vi "Digital - Continuous Input.vi"() -> ()   [LabVIEW 2014]
doc: "This example demonstrates how to acquire a continuous amount of digital data based off of a sample clock.\n\nSome hardware (e.g. M Series DAQ) must use an external sample clock for digital tasks. To view a complete list of available sample clock sources, consult the Device Routes table in Measurement and Automation Explorer.\n\nFor instructions on how to connect your signals to the DAQ device, refer to your device documentation."
uses:
  <vilib>/Utility/error.llb/DialogType.ctl
  <vilib>/DAQmx/read.llb/DAQmx Read (Digital Wfm 1Chan NSamp).vi
  <vilib>/DAQmx/create/channels.llb/DAQmx Create Channel (DI-Digital Input).vi
  <vilib>/DAQmx/configure/timing.llb/DAQmx Timing (Sample Clock).vi
  <vilib>/DAQmx/configure/trigger.llb/DAQmx Start Trigger (Digital Edge).vi
  <vilib>/DAQmx/configure/trigger.llb/DAQmx Reference Trigger (Digital Edge).vi
  <vilib>/DAQmx/miscellaneous.llb/DAQmx Fill In Error Info.vi
  <vilib>/Waveform/DWDTOps.llb/DWDT Digital to Binary U8.vi
  <resource>/objmgr/daqmx.rc
panel:
  in  "write to disk":bool
  in  "file path (use dialog)":path=path "e:/fire3.dat"
  in  "Samples per Loop":i32=100000
  in  "Stop":bool
  out "Digital Waveform Graph":digitalwaveform(graph)
  in  "Trigger Type":T1(tab)=enum."Digital Start"
  in  "Edge":i32(ring)=10280 items=["Rising"=10280, "Falling"=10171]
  in  "Digital Trigger Source":tag="/Dev1/PFI9"
  in  "Digital Trigger Source":tag="/Dev1/PFI9"
  in  "Edge":i32(ring)=10280 items=["Rising"=10280, "Falling"=10171]
  in  "pretrigger samples per channel":u32=2
  in  "Sample Rate":dbl=100000.0
  in  "Sample Clock Source":tag="OnboardClock"
  out "Actual Sample Rate":dbl=1000.0 format="%0.2f"
  in  "Line(s)":tag="Dev1/port0/line0:2"
  # "Channel Settings"
  # "Acquired Data"
  # "Timing Settings"
  # "Logging Settings"
  # "Trigger Settings"
  # "To configure and use a start trigger you must have the necessary tab selected above.  Not all hardware supports triggering--refer to your device documentation for more info."
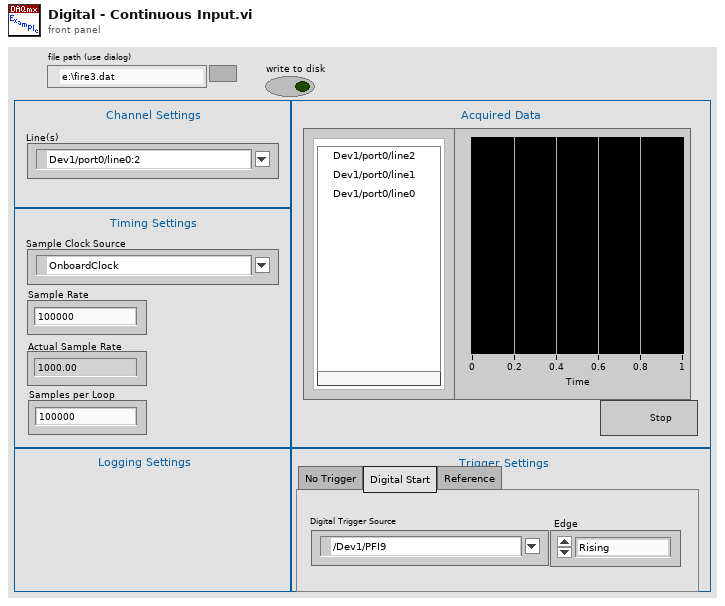
[diagram p1: front panel]
types:
  T1 = enum32{"No Trigger", "Digital Start", "Reference"}
  T2 = typedef "DialogType.ctl" = u16
  T3 = enum16{"big-endian, network order", "native, host order", "little-endian"}
  T4 = enum16{"open", "replace", "create", "open or create", "replace or create", "replace or create with confirmation"}
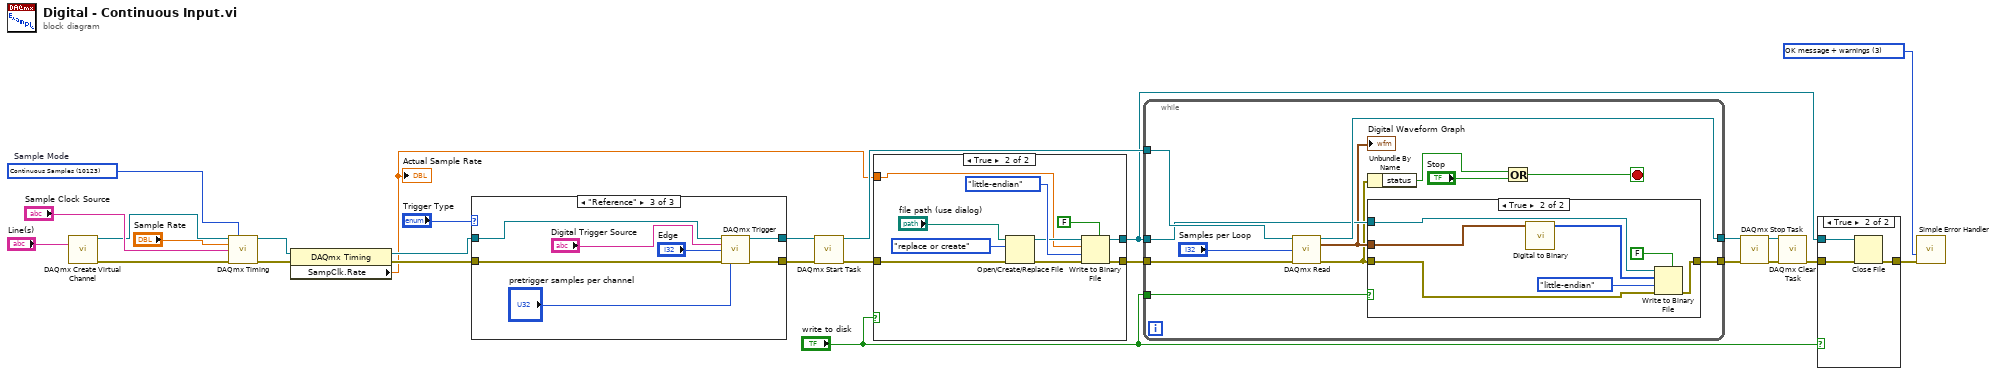
[diagram p0: block diagram]
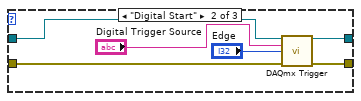
[diagram p6: hidden frame]
diagram:
  w10 = T2 3 items=["no dialog", "OK message", "continue or stop message", "OK message + warnings", "continue/stop + warnings"] ("type of dialog (OK msg:1)")
  w25 = 10123 items=["Finite Samples"=10178, "Continuous Samples"=10123, "Hardware Timed Single Point"=12522]  # Sample Mode
  n1 = call-poly <vilib>:"DAQmx Create Virtual Channel.vi"("lines"="Line(s)") -> ("task out"=w22:refnum<k21>, "error out"=w21:errorcluster)  [unwired: 13 in]
  n2 = call-poly <vilib>:"DAQmx Timing.vi"("task/channels in"=w22, "sample mode"=w25, "rate"="Sample Rate", "source"="Sample Clock Source", "error in"=w21) -> ("task out"=w20:refnum<k21>, "error out"=w19:errorcluster)  [unwired: 9 in]
  n3 = property class="DAQmx Timing"(reference=w20, error in=w19) -> (reference out=w8:refnum<k21>, error out=w9:errorcluster, "SampClk.Rate"=w1:dbl)
  "Actual Sample Rate" <- w1
  n4 = case shown="\"Reference\"" "Trigger Type" {
    tunnel: w8 -> [w28 w34 w41]
    tunnel: w9 -> [w27 w33 w40]
    tunnel: [w28 w32 w39] -> w17
    tunnel: [w27 w31 w38] -> w16
    frame "No Trigger", Default {
    }
    frame "Digital Start" {
      n5 = call-poly <vilib>:"DAQmx Trigger.vi"("task/channels in"=w34, "source"="Digital Trigger Source", "edge"="Edge", "error in"=w33) -> ("task out"=w32:refnum<k21>, "error out"=w31:errorcluster)  [unwired: 10 in]
    }
    frame "Reference" {
      n6 = call-poly <vilib>:"DAQmx Trigger.vi"("task/channels in"=w41, "source"="Digital Trigger Source", "edge"="Edge", "error in"=w40, "pretrigger samples per channel"="pretrigger samples per channel") -> ("task out"=w39:refnum<k21>, "error out"=w38:errorcluster)  [unwired: 9 in]
    }
  }
  n7 = call <vilib>:"DAQmx Start Task.vi"("task/channels in"=w17, "error in"=w16) -> ("task out"=w15:refnum<k21>, "error out"=w4:errorcluster)  [unwired: 12 in]
  n8 = case shown="True" "write to disk" {
    tunnel: [_ w46] -> w5
    tunnel: w4 -> [w42 w50]
    tunnel: [w42 w44] -> w3
    tunnel: w1 -> [_ w43]
    frame False {
    }
    frame True {
      n9 = Open/Create/Replace File(file path (use dialog)="file path (use dialog)", error in=w50, operation (0:open)=T4."replace or create") -> (refnum out=w47:refnum<file>, error out=w45:errorcluster)  [unwired: 3 in, 1 out]
      n10 = Write to Binary File(file (use dialog)=w47, data=w43, error in=w45, 5:FALSE ("prepend array or string size? (T)"), 9:T3."little-endian" ("byte order (0:big-endian, network order)")) -> (refnum out=w46:refnum<file>, error out=w44:errorcluster)  [unwired: 1 in, 1 out]
    }
  }
  n11 = while {
    tunnel: [w64] -> w12
    tunnel: [w54] -> w11
    tunnel: w3 -> [w63]
    tunnel: w15 -> [w62]
    tunnel: w5 -> [w57]
    tunnel: "write to disk" -> [w53]
    stop <- w59 stop-if-true
    n12 = call-poly <vilib>:"DAQmx Read.vi"("task/channels in"=w62, "number of samples per channel"="Samples per Loop", "error in"=w63) -> ("task out"=w64:refnum<k21>, "data"=w56:digitalwaveform, "error out"=w55:errorcluster)  [unwired: 10 in]
    "Digital Waveform Graph" <- w56
    n13 = Unbundle By Name(w55) -> ("status"=w61:bool)
    n14 = case shown="True" w53 {
      tunnel: w57 -> [_ w67]
      tunnel: w56 -> [_ w72]
      tunnel: w55 -> [w65 w66]
      tunnel: [w65 w70] -> w54
      frame False {
      }
      frame True {
        n15 = call-poly <vilib>:"Digital to Binary.vi"("digital waveform"=w72) -> ("binary array"=w71:u8[])  [unwired: 9 in, 1 out]
        n16 = Write to Binary File(file (use dialog)=w67, data=w71, error in=w66, 5:FALSE ("prepend array or string size? (T)"), 9:T3."little-endian" ("byte order (0:big-endian, network order)")) -> (error out=w70:errorcluster)  [unwired: 1 in, 2 out]
      }
    }
    n17 = Or(x=w61, y="Stop") -> (x .or. y?=w59:bool)
  }
  n18 = call <vilib>:"DAQmx Stop Task.vi"("task/channels in"=w12, "error in"=w11) -> ("task out"=w14:refnum<k21>, "error out"=w13:errorcluster)  [unwired: 12 in]
  n19 = call <vilib>:"DAQmx Clear Task.vi"("task in"=w14, "error in"=w13) -> ("error out"=w7:errorcluster)  [unwired: 13 in]
  n20 = case shown="True" "write to disk" {
    tunnel: w7 -> [w73 w76]
    tunnel: [w73 w75] -> w6
    tunnel: w5 -> [_ w74]
    frame False {
    }
    frame True {
      n21 = Close File(refnum=w74, error in=w76) -> (error out=w75:errorcluster)  [unwired: 1 out]
    }
  }
  n22 = call <vilib>:"Simple Error Handler.vi"("type of dialog (OK msg:1)"=w10, "error in (no error)"=w6) -> ()  [unwired: 3 in, 5 out]
